vi "_MainOpenMV_New.vi"(11 "Port":string) -> (2 "Script Out":string)   [LabVIEW 2022 SP3]
uses:
  Processors.ctl
  _subs/CameraSetup.ctl
panel:
  in  "Make Main":bool
  out "ROI":T1={"left"=0, "top"=0, "right"=320, "bottom"=240}
  in  "Set ROI":bool
  out "roi":string
  in  "Set Threshold":bool
  in  "clear":bool
  out "Plots":T2
  out "Lab":string="[10,90,-40,40,-40,40]"
  out "Tx Buffer":string
  in  "Play":bool
  in  "Serial Port":string(combo)="ASRL30::INSTR"
  out "Version":string
  in  "Connect":bool
  out "FPS":dbl format="%#.2g"
  in  "Tabs":enum32{"Simple View", "REPL", "Python"}(tab)
  in  "Destination Info":enum32{"None", "UART", "SPI", "I2C", "WiFi"}(tab)
  in  "WiFi Info":T3={"WiFi"={"SSID"="", "Key"=""}, "SystemLink"={"APIKey"="", "Tag"="", "Type"="STRING"}}
  in  "Destination":enum16{"None", "UART", "SPI", "I2C", "WiFi"}(ring)
  out "Value":dbl(graph)
  in  "View":T4(ring)=enum."Nothing"
  in  "Params":T5(tab)
  in  "Color Statistic":u16(ring) items=["l_mean", "l_median", "l_mode", "l_sdev", "l_min", "l_max", "l_lower quartile", "l_upper quartile", "a_mean", "a_median", "a_mode", "a_sdev", "a_min", "a_max", "a_lq", "a_uq", "b_mean", "b_median", "b_mode", "b_sdev", "b_max", "b_min", "b_lq", "b_uq", "All statistics"]
  in  "Gray Statistic":u16(ring)=1 items=["mean", "median", "mode", "sdev", "min", "max", "lower quartile", "upper quartile", "All statistics"]
  in  "Blob Params":T6={"B[0]_Feature"=enum."# blobs", "Lab thresholds"="[10,90,-20,20,-20,20]", "Min Pixels"=100, "Min Area (box)"=100, "Merge"=TRUE, "Margin for merge"=10}
  in  "Face Parameter":u16(ring) items=["# faces", "All data"]
  in  "QR Return":u16(ring)=4 items=["x", "y", "w", "h", "payload", "version", "ecc_level", "mask", "data_type", "All data"]
  in  "Ctrl D":bool
  in  "Grab Script":bool
  in  "Line":u8(slide) scale=0.0..25.0
  in  "Send Line":bool
  out "Console":string
  in  "Notepad":string
  in  "Ctrl C":bool
  out "rows":string="  1\n  2\n  3\n  4\n  5\n  6\n  7\n  8\n  9\n 10\n 11\n 12\n 13\n 14\n 15\n 16\n 17\n 18\n 19\n 20\n 21\n"
  in  "Script":string="# Show Color - lmean\n\nimport sensor, image, time\n\nsensor.reset()\nsensor.set_pixformat(sensor.RGB565)\nsensor.set_framesize(sensor.QVGA)\nsensor.skip_frames(time = 2000)\n\nsensor.set_auto_gain(False)\nsensor.set_auto_whitebal(False) \n\nclock = time.clock()\n\n\n\nwhile(True):\n    clock.tick()\n    img = sensor.snapshot()\n    \n    print(img.statistics()[0])\n"
  in  "New":bool
  in  "Load":bool
  in  "Save":bool
  in  "File":path
  in  "startCode":string
  out "Size":string
  in  "stop":bool
  out "image":picture
  # "LabVIEW OpenMV"
  # "Note: i2c and SPI and WiFi are having issues"
  # "Use P4 for Tx and P5 for Rx and GND for ground\n\nDefault BAUD rate is 19200 - you can change this\nby editing the Python code (Python tab)"
  # "Use P0 for MOSI, P1 for MISO, P2 for SCLK, P3 for SS (active low)\n and GND for ground\n\nThe default is being an SPI slave - note that you can miss data\nin this mode"
  # "Use P4 for SCL and P5 for SDA and GND for ground\n\nThis runs as an i2c slave"
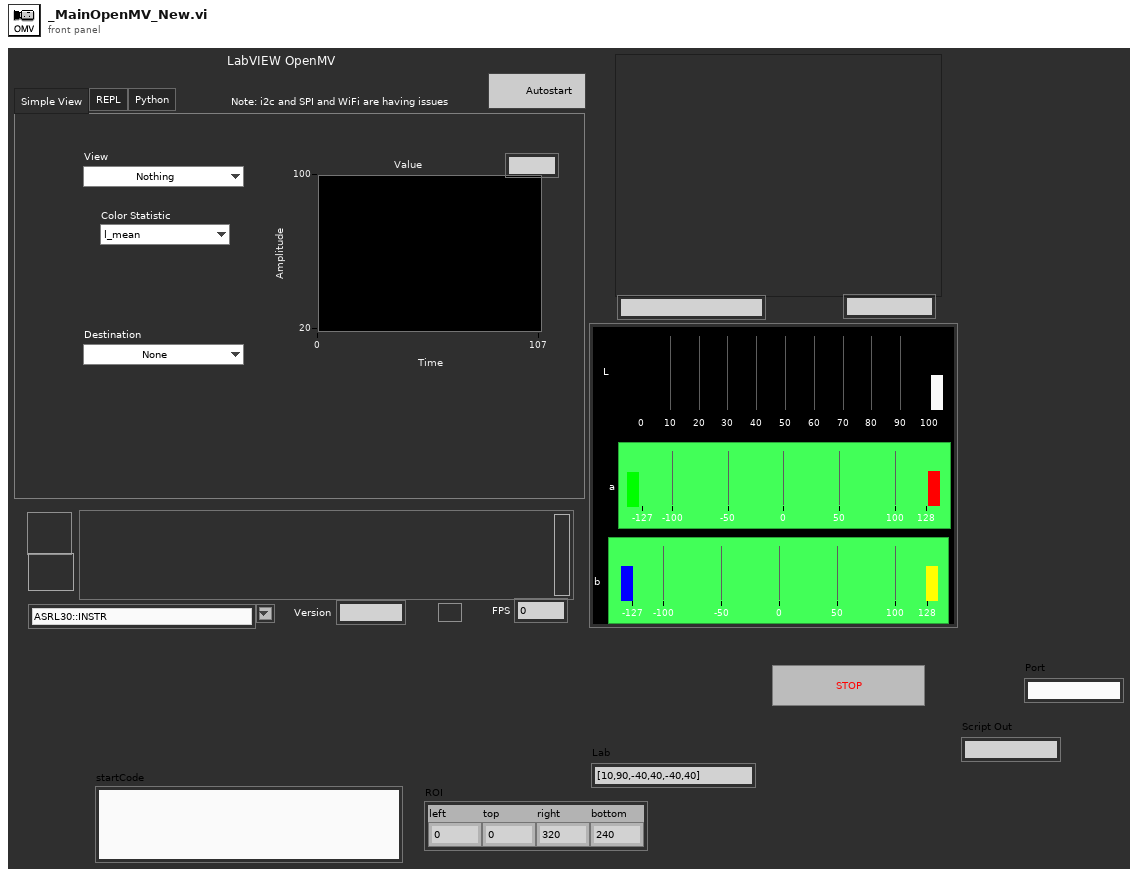
[diagram p1: front panel]
types:
  T1 = cluster{"left":i16, "top":i16, "right":i16, "bottom":i16}
  T2 = cluster{"L":dbl[], "a":cluster{i32, i32, dbl[]}, "b":cluster{i32, i32, dbl[]}}
  T3 = cluster{"WiFi":cluster{"SSID":string, "Key":string}, "SystemLink":cluster{"APIKey":string, "Tag":string, "Type":string}}
  T4 = enum16{"Color stats", "Nothing", "Greyscale stats", "Track Blobs", "Track Faces", "QRCode"}
  T5 = enum32{"C_ Stat", "G_Stats", "Blobs", "Face", "QR"}
  T6 = cluster{"B[0]_Feature":enum16{"x", "y", "width", "height", "pixels", "cx", "cy", "rotation", "code", "count", "# blobs", "All parameters"}, "Lab thresholds":string, "Min Pixels":i16, "Min Area (box)":i16, "Merge":bool, "Margin for merge":i16}
  T7 = typedef "Processors.ctl" = enum16{"SPIKE", "Pi", "Pi_ssh", "OpenMV", "Dunio"}
  T8 = enum8{"Enabled", "Disabled", "Disabled and Grayed Out"}
  T9 = enum16{"Color stats", "Greyscale stats", "Track Blobs", "Track Faces", "QRCode"}
  T10 = typedef "CameraSetup.ctl" = cluster{"Format":enum16{"GRAYSCALE", "RGB565", "BAYER"}, "size":enum16{"QQQQVGA (40x30)", "QQQVGA (80x60)", "QQVGA (160x120)", "QVGA (320x240)", "VGA (640x480)", "LCD (128x160)", "B64x32 (64x32)", "B64x64", "B128x64", "B128x128"}, "Skip frames (ms)":u16, "autoGain":bool, "autoWhitebal":bool}
  T11 = typedef "PythonCtrl.ctl" = cluster{"session":refnum<k35>, "PyPath":path, "Processor":T7, "Port":string, "version":string}
  T12 = typedef "imagedata.ctl" = cluster{"image type":i32, "image depth":i32, "image":u8[], "mask":u8[], "colors":u32[], "Rectangle":cluster{"left":i16, "top":i16, "right":i16, "bottom":i16}}
  T13 = typedef "Preferences.ctl" = cluster{"python":string, "arduino CLI":path, "pythonCodes":cluster{"pythonCode":path, "Color":u32}[], "FontSize":u8, "Text Colors":cluster{"Quote":u32, "function":u32, "Python":u32, "Comment":u32, "Triple Quote":u32, "Text":u32}, "SSH Logins":cluster{"IP Address":string, "Username":string, "password":string}[], "packet size":u8}
  T14 = cluster{"left":i32, "top":i32, "right":i32, "bottom":i32}
  T15 = typedef "eventvkey.ctl" = enum16{"ASCII", "Enter", "Return", "Shift", "Ctrl", "Alt", "Cmd", "Opt", "Caps", "NumLock", "Clear", "Break", "Up", "Down", "Left", "Right", "Insert", "Delete", "Home", "End", "PageUp", "PageDown", "Escape", "Help", "Pause", "ScrollLock", "F1", "F2", "F3", "F4", "F5", "F6", "F7", "F8", "F9", "F10", "F11", "F12", "F13", "F14", "F15", "F16", "F17", "F18", "F19", "F20", "F21", "F22", "F23", "F24", "Play", "VolumeUp", "VolumeDown", "Mute", "Two Byte Char"}
  T16 = cluster{"Shift":bool, "Ctrl":bool, "Alt":bool, "Cmd":bool, "Opt":bool}
  T17 = cluster{"Char":i16, "VKey":T15, "ScanCode":i16, "Mods":cluster{"Num Pad":bool, "Menu Key":bool}, "PlatMods":cluster{"Shift":bool, "Ctrl":bool, "Alt":bool, "Cmd":bool, "Opt":bool}, "FocusObj":refnum<vi>}
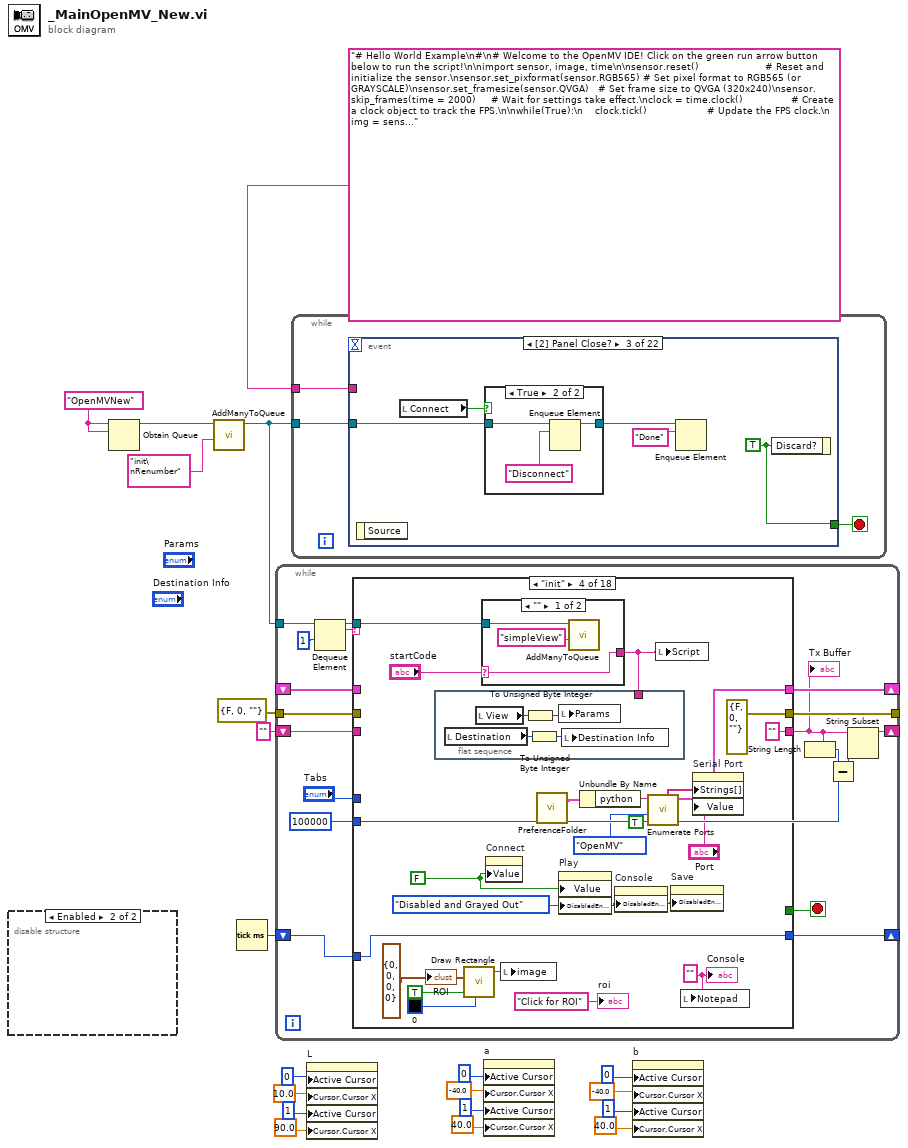
[diagram p0: block diagram]
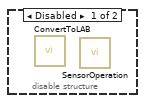
[diagram p2: hidden frame]
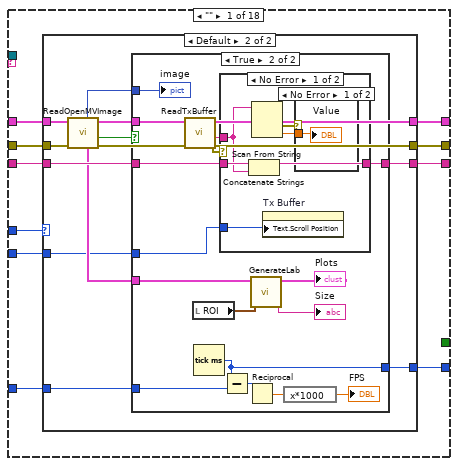
[diagram p3: hidden frame]
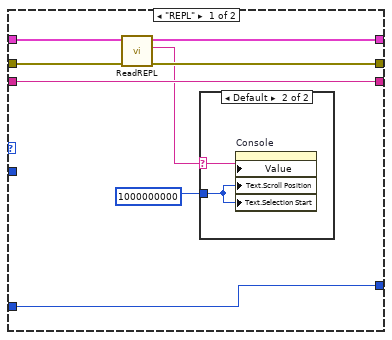
[diagram p4: hidden frame]
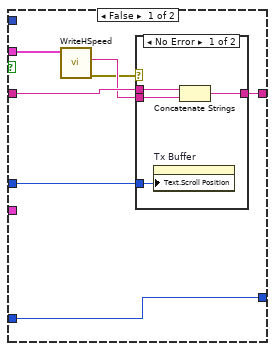
[diagram p6: hidden frame]
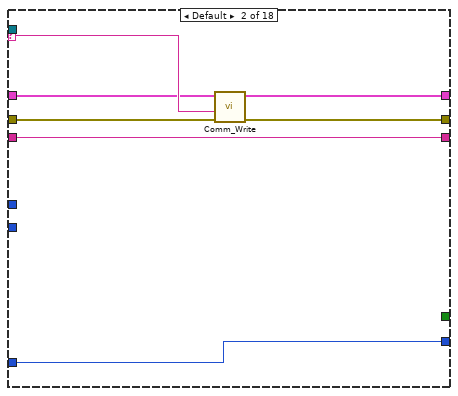
[diagram p10: hidden frame]
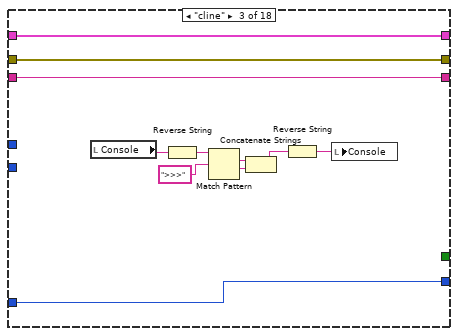
[diagram p11: hidden frame]
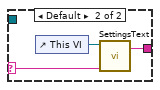
[diagram p12: hidden frame]
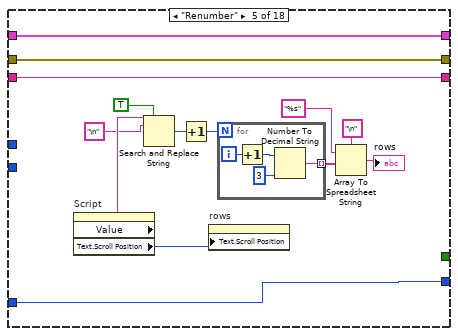
[diagram p13: hidden frame]
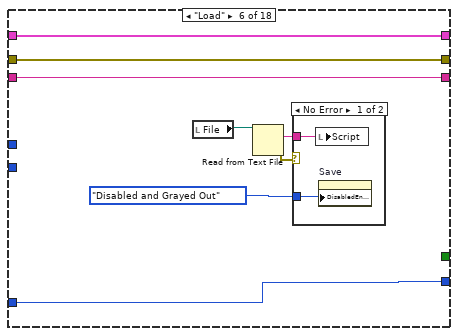
[diagram p14: hidden frame]
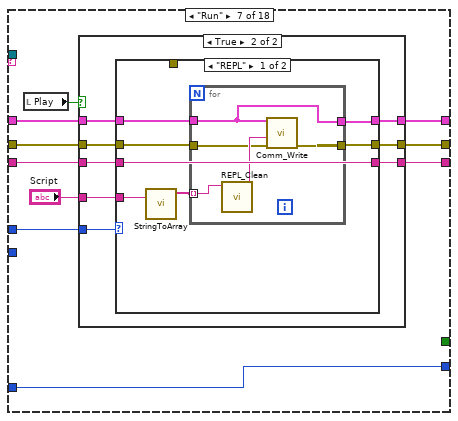
[diagram p16: hidden frame]
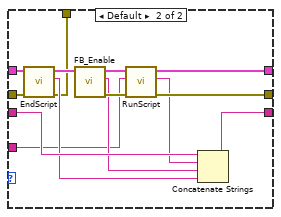
[diagram p18: hidden frame]
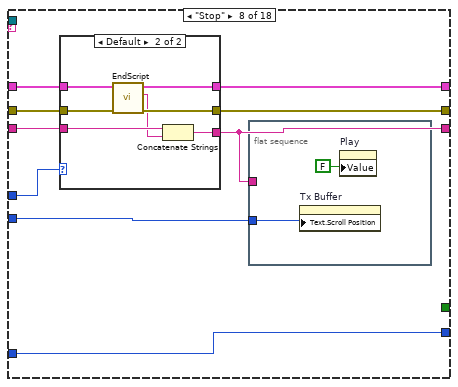
[diagram p19: hidden frame]
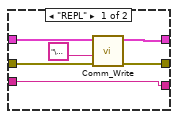
[diagram p20: hidden frame]
diagram:
  w20 = "OpenMVNew" ("name (unnamed)")
  n1 = disable-structure shown="Enabled" {
    frame Disabled {
      n2 = call "ConvertToLAB.vi"() -> ()  [unwired: 9 in, 3 out]
      n3 = call "SensorOperation.vi"() -> ()  [unwired: 11 in, 1 out]
    }
    frame Enabled {
    }
  }
  n4 = Obtain Queue(name (unnamed)=w20, element data type=w20) -> (queue out=w15:refnum<queue>)  [unwired: 3 in, 2 out]
  n5 = call "AddManyToQueue.vi"("Cmds"="init\nRenumber", "Queue in"=w15) -> ("Queue out"=w17:refnum<queue>)  [unwired: 9 in]
  n6 = Tick Count (ms)() -> (millisecond timer value=w18:u32)
  n7 = while {
    tunnel: w17 -> [w37]
    shift-right: [w34] -> _
    shift-left: _ -> [w35]
    shift-right: [w28] -> _
    shift-left: "" ("Tx Buffer") -> [w27]
    tunnel: errorcluster {"status"=FALSE, "code"=0, "source"=""} ("error out") -> [w32]
    tunnel: [w31] -> _
    shift-right: [w30] -> _
    shift-left: w18 -> [w29]
    stop <- w33 stop-if-true
    w25 = 100000 ("length (rest)")
    n8 = Dequeue Element(queue=w37, timeout in ms (-1)=1) -> (queue out=w21:refnum<queue>, element=w36:string)  [unwired: 1 in, 2 out]
    n9 = case shown="\"init\"" w36 {
      selector: w36 -> [_ w110 _ _ _ _ _ _ _ _ _ _ _ _ _ _ _ _]
      tunnel: w35 -> [w48 w107 w121 _ w168 w180 w192 w238 w261 w267 w307 w322 w346 w354 w366 w432 w437 w445]
      tunnel: [w45 w107 w121 w125 w168 w180 w190 w235 w258 w276 w298 w322 w346 w354 w366 w432 w437 w445] -> w34
      tunnel: [w46 w108 w120 errorcluster {"status"=FALSE, "code"=0, "source"=""} ("error out") w167 w179 w189 w236 w259 w275 w305 w321 w345 w353 w378 w431 w438 w444] -> w31
      tunnel: w32 -> [w47 w109 w120 _ w167 w179 w191 w237 w260 w274 w306 w321 w345 w353 w378 w431 w438 w444]
      tunnel: w27 -> [w44 w112 w123 _ w166 w178 w188 w233 w256 w273 w308 w320 w344 w352 w380 _ w435 w443]
      tunnel: [w43 w112 w123 "" ("Tx Buffer") w166 w178 w187 w231 w254 w273 w308 w320 w344 w352 w380 "" ("Tx Buffer") w434 w443] -> w24
      tunnel: [_ _ _ _ _ _ _ _ _ _ _ _ _ _ _ _ _ TRUE] -> w33
      tunnel: [w42 w111 w122 w142 w165 w177 w186 w234 w257 w272 w303 w318 w343 w351 w379 w433 w439 w441] -> w30
      tunnel: w29 -> [w41 w111 w122 w142 w165 w177 w186 w234 w257 w272 w303 w318 w343 w351 w379 w433 w439 w441]
      tunnel: w25 -> [w40 _ _ _ _ _ _ w232 w255 _ w299 _ _ _ _ _ _ _]
      tunnel: "Tabs" -> [w39 _ _ _ _ _ w184 w230 _ _ _ _ _ _ _ _ _ _]
      tunnel: w21 -> [_ _ _ w131 _ _ _ _ _ _ _ _ _ _ _ _ _ _]
      frame "" {
        n10 = case shown="Default" w39 {
          tunnel: w48 -> [w56 w68]
          tunnel: w47 -> [w55 w67]
          tunnel: [w53 w66] -> w46
          tunnel: [w54 w65] -> w45
          tunnel: w44 -> [w52 w64]
          tunnel: [w52 w63] -> w43
          tunnel: [w51 w62] -> w42
          tunnel: w41 -> [w51 w61]
          tunnel: w40 -> [_ w59]
          frame "REPL" {
            n11 = call "ReadREPL.vi"("error in (no error)"=w55, "Python"=w56) -> ("error out"=w53:errorcluster, "String"=w49:string, "Python"=w54:T11)  [unwired: 6 in, 1 out]
            n12 = case shown="Default" w49 {
              selector: w49 -> [_ w57]
              tunnel: u32 1000000000 ("Text.Selection:Start") -> [_ w58]
              frame "" {
              }
              frame Default {
                n13 = property on="Console" class="Str"("Value"=w57, "Text.Scroll Position"=w58, "Text.Selection Start"=w58) -> ()  [unwired: 2 in, 2 out]
              }
            }
          }
          frame Default {
            n14 = call "ReadOpenMVImage.vi"("error in"=w67, "Python"=w68) -> ("error out"=w66:errorcluster, "Good?"=w70:bool, "Python"=w65:T11, "image data"=w60:T12, "new picture"=w69:picture)  [unwired: 4 in, 1 out]
            n15 = case shown="True" w70 {
              tunnel: w69 -> [_ w92]
              tunnel: w65 -> [w73 w98]
              tunnel: [w75 w88] -> w63
              tunnel: w64 -> [w76 w86]
              tunnel: [w77 w97] -> w62
              tunnel: w61 -> [w77 w96]
              tunnel: w60 -> [_ w90]
              tunnel: w59 -> [w74 w83]
              frame False {
                n16 = call "WriteHSpeed.vi"("Python"=w73) -> ("error out"=w71:errorcluster, "read buffer"=w72:string)  [unwired: 8 in, 1 out]
                n17 = case shown="No Error" w71 {
                  tunnel: w72 -> [w81 _]
                  tunnel: w76 -> [w80 w82]
                  tunnel: [w79 w82] -> w75
                  tunnel: w74 -> [w78 _]
                  frame No Error {
                    n18 = property on="Tx Buffer" class="Str"("Text.Scroll Position"=w78) -> ()  [unwired: 2 in, 2 out]
                    n19 = Concatenate Strings(w80, w81) -> (w79:string)
                  }
                  frame Error {
                  }
                }
              }
              frame True {
                n20 = call "ReadTxBuffer.vi"("Python"=w98) -> ("error out"=w84:errorcluster, "Tx Buffer"=w85:string)  [unwired: 7 in, 2 out]
                n21 = local read "ROI"() -> (w89:T1)
                n22 = Tick Count (ms)() -> (millisecond timer value=w97:u32)
                n23 = case shown="No Error" w84 {
                  tunnel: [w104 w106] -> w88
                  tunnel: w86 -> [w101 w106]
                  tunnel: w85 -> [w100 _]
                  tunnel: w83 -> [w99 _]
                  frame No Error {
                    n24 = Concatenate Strings(w101, w100) -> (w104:string)
                    n25 = Scan From String(input string=w100) -> (error out=w103:errorcluster, output 1=w102:dbl)  [unwired: 4 in, 2 out]
                    n26 = property on="Tx Buffer" class="Str"("Text.Scroll Position"=w99) -> ()  [unwired: 2 in, 2 out]
                    n27 = case shown="No Error" w103 {
                      tunnel: w102 -> [w105 _]
                      frame No Error {
                        "Value" <- w105
                      }
                      frame Error {
                      }
                    }
                  }
                  frame Error {
                  }
                }
                n28 = Subtract(x=w97, y=w96) -> (x-y=w93:u32)
                n29 = Reciprocal(x=w93) -> (1/x=w95:dbl)
                n30 = call "GenerateLab.vi"("ROI"=w89, "image data"=w90) -> ("Dimensions"=→"Size":string, "Plots"=→"Plots":T2)  [unwired: 8 in]
                n31 = expression code="x*1000"(w95) -> (→"FPS":dbl)
                "image" <- w92
              }
            }
          }
        }
      }
      frame Default {
        n32 = call "Comm_Write.vi"("error in (no error)"=w109, "Text to write"=w110, "Python"=w107) -> ("error out"=w108:errorcluster)  [unwired: 7 in, 1 out]
      }
      frame "cline" {
        n33 = local read "Console"() -> (w113:string)
        n34 = Reverse String(1:w113) -> (0:w119:string)
        n35 = Match Pattern(string=w119, regular expression=">>>") -> (match substring=w116:string, after substring=w117:string)  [unwired: 1 in, 2 out]
        n36 = Concatenate Strings(w116, w117) -> (w115:string)
        n37 = Reverse String(1:w115) -> (0:w114:string)
        n38 = local write "Console"(w114) -> ()
      }
      frame "init" {
        w137 = "" ("Tx Buffer")
        w135 = T1 {"left"=0, "top"=0, "right"=0, "bottom"=0} ("rect")
        w136 = T8."Disabled and Grayed Out" ("Disabled")
        w138 = FALSE ("Connect")
        n39 = flat-sequence {
          tunnel: w132 -> [_]
          frame #0 {
            n40 = local read "Destination"() -> (w151:enum16{"None", "UART", "SPI", "I2C", "WiFi"})
            n41 = local read "View"() -> (w154:T4)
            n42 = To Unsigned Byte Integer(number=w154) -> (unsigned 8bit integer=w153:u8)
            n43 = To Unsigned Byte Integer(number=w151) -> (unsigned 8bit integer=w152:u8)
            n44 = local write "Params"(w153) -> ()
            n45 = local write "Destination Info"(w152) -> ()
          }
        }
        n46 = call <vilib>:"Draw Rectangle.vi"("rect"=w135, "fill?(F)"=TRUE, "color(black)"=u32 0) -> ("new picture"=w139:picture)  [unwired: 6 in]
        n47 = case shown="\"\"" "startCode" {
          selector: "startCode" -> [w147 w148]
          tunnel: [w147 w149] -> w132
          tunnel: w131 -> [w146 _]
          frame "" {
            n48 = call "AddManyToQueue.vi"("Cmds"="simpleView", "Queue in"=w146) -> ()  [unwired: 9 in, 1 out]
          }
          frame Default {
            n49 = control-ref of="This VI"() -> (w150:refnum<vi>)
            n50 = call "SettingsText.vi"("Saved code"=w148, "VI in"=w150) -> ("Python Code out"=w149:string)  [unwired: 8 in, 1 out]
          }
        }
        n51 = property on="Connect" class="Bool (strict)"("Value"=w138) -> ()  [unwired: 2 in, 2 out]
        n52 = local write "image"(w139) -> ()
        n53 = call "PreferenceFolder.vi"() -> ("Everything"=w126:T13)  [unwired: 4 in, 7 out]
        n54 = property on="Play" class="Bool (strict)"("Value"=w138, "DisabledEnum"=w136) -> ()  [unwired: 2 in, 2 out]
        n55 = Unbundle By Name(w126) -> ("python"=w129:string)
        n56 = property on="Console" class="Str"("DisabledEnum"=w136) -> ()  [unwired: 2 in, 2 out]
        n57 = call "Enumerate Ports.vi"("list?"=TRUE, "Processor"=Processors."OpenMV", "Python version"=w129) -> ("Python"=w125:T11, "possibilities"=w130:string[])  [unwired: 3 in, 4 out]
        n58 = local write "Script"(w132) -> ()
        n59 = property on="Save" class="Bool"("DisabledEnum"=w136) -> ()  [unwired: 2 in, 2 out]
        n60 = local write "Notepad"(w137) -> ()
        n61 = property on="Serial Port" class="CmbBox"("Strings[]"=w130, "Value"="Port") -> ()  [unwired: 2 in, 2 out]
        "Console" <- w137
        "roi" <- "Click for ROI" ("roi")
        "ROI" <- w135
      }
      frame "Renumber" {
        n62 = property on="Script" class="Str"() -> ("Value"=w164:string, "Text.Scroll Position"=w163:u32)  [unwired: 2 in, 2 out]
        n63 = Search and Replace String(replace all?=TRUE ("replace all? (F)"), input string=w164, search string="\n") -> (number of replacements=w162:i32)  [unwired: 5 in, 3 out]
        n64 = Increment(x=w162) -> (x+1=w155:i32)
        n65 = property on="rows" class="Str"("Text.Scroll Position"=w163) -> ()  [unwired: 2 in, 2 out]
        n66 = for {
          N: w155 -> [_]
          tunnel: [w172] -> w160 mode=indexing
          i -> [w169]
          n67 = Increment(x=w169) -> (x+1=w171:i32)
          n68 = Number To Decimal String(number=w171, width (-)=i16 3) -> (decimal integer string=w172:string)
        }
        n69 = Array To Spreadsheet String(delimiter (Tab)="\n", array=w160, 3:"%s" ("format string")) -> (spreadsheet string=→"rows":string)
      }
      frame "Load" {
        n70 = local read "File"() -> (w176:path)
        n71 = Read from Text File(file (use dialog)=w176) -> (text=w173:string, error out=w174:errorcluster)  [unwired: 3 in, 2 out]
        n72 = case shown="No Error" w174 {
          tunnel: T8."Disabled and Grayed Out" ("Disabled") -> [w182 _]
          tunnel: w173 -> [w181 _]
          frame No Error {
            n73 = local write "Script"(w181) -> ()
            n74 = property on="Save" class="Bool"("DisabledEnum"=w182) -> ()  [unwired: 2 in, 2 out]
          }
          frame Error {
          }
        }
      }
      frame "Run" {
        n75 = local read "Play"() -> (w185:bool)
        n76 = case shown="True" w185 {
          tunnel: w192 -> [w195 w203]
          tunnel: w191 -> [w194 w202]
          tunnel: [w195 w201] -> w190
          tunnel: [w194 w200] -> w189
          tunnel: w188 -> [w193 w198]
          tunnel: [w193 w199] -> w187
          tunnel: w184 -> [_ w197]
          tunnel: "Script" -> [_ w196]
          frame False {
          }
          frame True {
            n77 = case shown="\"REPL\"" w197 {
              tunnel: w203 -> [w209 w226]
              tunnel: w202 -> [w208 w225]
              tunnel: [w206 w224] -> w201
              tunnel: [w207 w223] -> w200
              tunnel: [w204 w222] -> w199
              tunnel: w198 -> [w204 w221]
              tunnel: w196 -> [w205 w217]
              tunnel: [_ w216] -> _
              frame "REPL" {
                n78 = call "StringToArray.vi"("write buffer"=w205) -> ("Array"=w210:string[])  [unwired: 10 in]
                n79 = for {
                  tunnel: w210 -> [w215] mode=indexing
                  tunnel: w209 -> [w211]
                  tunnel: w208 -> [w213]
                  tunnel: [w212] -> w207
                  tunnel: [w211] -> w206
                  n80 = call "REPL_Clean.vi"("Code in"=w215) -> ("Code cleaned"=w214:string)  [unwired: 10 in]
                  n81 = call "Comm_Write.vi"("error in (no error)"=w213, "Text to write"=w214, "Python"=w211) -> ("error out"=w212:errorcluster)  [unwired: 7 in, 1 out]
                }
              }
              frame Default {
                n82 = call "EndScript.vi"("error in (no error)"=w225, "Python"=w226) -> ("error out"=w216:errorcluster, "Tx for stopping code"=w218:string, "Python"=w229:T11)  [unwired: 7 in]
                n83 = call "FB_Enable.vi"("Python"=w229) -> ("error out"=w228:errorcluster, "Reply"=w219:string, "Python"=w227:T11)  [unwired: 8 in]
                n84 = call "RunScript.vi"("error in"=w228, "script"=w217, "Python"=w227) -> ("error out"=w223:errorcluster, "Tx"=w220:string, "Python"=w224:T11)  [unwired: 6 in]
                n85 = Concatenate Strings(w221, w220, w219, w218) -> (w222:string)
              }
            }
          }
        }
      }
      frame "Stop" {
        n86 = case shown="Default" w230 {
          tunnel: w238 -> [w239 w250]
          tunnel: w237 -> [w242 w249]
          tunnel: [w240 w248] -> w236
          tunnel: [w239 w247] -> w235
          tunnel: w233 -> [w243 w246]
          tunnel: [w243 w244] -> w231
          frame "REPL" {
            n87 = call "Comm_Write.vi"("error in (no error)"=w242, "Text to write"="\u0003" ("write buffer"), "Python"=w239) -> ("error out"=w240:errorcluster)  [unwired: 7 in, 1 out]
          }
          frame Default {
            n88 = call "EndScript.vi"("error in (no error)"=w249, "Python"=w250) -> ("error out"=w248:errorcluster, "Tx for stopping code"=w245:string, "Python"=w247:T11)  [unwired: 7 in]
            n89 = Concatenate Strings(w246, w245) -> (w244:string)
          }
        }
        n90 = flat-sequence {
          tunnel: w232 -> [w252]
          tunnel: w231 -> [_]
          frame #0 {
            n91 = property on="Tx Buffer" class="Str"("Text.Scroll Position"=w252) -> ()  [unwired: 2 in, 2 out]
            n92 = property on="Play" class="Bool (strict)"("Value"=FALSE ("Play")) -> ()  [unwired: 2 in, 2 out]
          }
        }
      }
      frame "stopForREPL" {
        n93 = call "EndScript.vi"("error in (no error)"=w260, "Python"=w261) -> ("error out"=w259:errorcluster, "Tx for stopping code"=w253:string, "Python"=w258:T11)  [unwired: 7 in]
        n94 = Concatenate Strings(w256, w253) -> (w254:string)
        n95 = flat-sequence {
          tunnel: w255 -> [w263]
          tunnel: w254 -> [_]
          frame #0 {
            n96 = property on="Tx Buffer" class="Str"("Text.Scroll Position"=w263) -> ()  [unwired: 2 in, 2 out]
            n97 = property on="Play" class="Bool (strict)"("Value"=FALSE ("Play")) -> ()  [unwired: 2 in, 2 out]
          }
        }
      }
      frame "Connect" {
        n98 = local read "Tabs"() -> (w269:enum32{"Simple View", "REPL", "Python"})
        n99 = Match Pattern(string="Serial Port", regular expression=":") -> (before substring=w265:string)  [unwired: 1 in, 3 out]
        n100 = Not Equal?(x=w269, y=enum32{"Simple View", "REPL", "Python"}."REPL") -> (x != y?=w271:bool)
        n101 = call "HighSpeedInit.vi"("error in"=w274, "Port"=w265, "Fast"=w271, "Python"=w267) -> ("error out"=w268:errorcluster, "Python"=w277:T11)  [unwired: 6 in]
        n102 = case shown="Error" w268 {
          selector: w268 -> [w278 w297]
          tunnel: w277 -> [w283 w294]
          tunnel: [w282 w294] -> w276
          tunnel: [w281 w297] -> w275
          tunnel: w269 -> [w280 _]
          frame No Error {
            w279 = T8."Enabled" ("Disabled")
            n103 = property on="Play" class="Bool (strict)"("DisabledEnum"=w279) -> ()  [unwired: 2 in, 2 out]
            n104 = case shown="\"REPL\"" w280 {
              tunnel: w278 -> [w287 w293]
              tunnel: w283 -> [w285 w292]
              tunnel: [w285 w290] -> w282
              tunnel: [w286 w289] -> w281
              tunnel: w279 -> [w288 _]
              frame "REPL" {
                n105 = property on="Console" class="Str"("DisabledEnum"=w288) -> ()  [unwired: 2 in, 2 out]
                n106 = call "Comm_Write.vi"("error in (no error)"=w287, "Text to write"="\n\n" ("write buffer"), "Python"=w285) -> ("error out"=w286:errorcluster)  [unwired: 7 in, 1 out]
              }
              frame Default {
                n107 = call "AskVersion.vi"("error in"=w293, "Python"=w292) -> ("error out"=w289:errorcluster, "Version"=→"Version":string, "Python"=w290:T11)  [unwired: 7 in]
              }
            }
          }
          frame Error {
            n108 = local write "Connect"(FALSE ("Connect")) -> ()
            n109 = One Button Dialog(message="Cannot initialize port. Try another") -> ()  [unwired: 1 in, 1 out]
          }
        }
      }
      frame "Disconnect" {
        w300 = T8."Disabled and Grayed Out" ("Disabled")
        n110 = local read "Tabs"() -> (w301:enum32{"Simple View", "REPL", "Python"})
        n111 = property on="Tx Buffer" class="Str"("Text.Scroll Position"=w299) -> ()  [unwired: 2 in, 2 out]
        n112 = case shown="Default" w301 {
          tunnel: [w310 w314] -> w298
          tunnel: w307 -> [w310 w313]
          tunnel: w306 -> [w309 w312]
          tunnel: [w309 w311] -> w305
          frame "REPL" {
          }
          frame Default {
            n113 = call "EndScript.vi"("error in (no error)"=w312, "Python"=w313) -> ("error out"=w311:errorcluster, "Python"=w314:T11)  [unwired: 7 in, 1 out]
          }
        }
        n114 = call "CloseHS.vi"("error in (no error)"=w305, "Python"=w298) -> ()  [unwired: 10 in]
        n115 = local write "Connect"(FALSE ("Connect")) -> ()
        n116 = property on="Play" class="Bool (strict)"("Value"=FALSE ("Play"), "DisabledEnum"=w300) -> ()  [unwired: 2 in, 2 out]
        n117 = property on="Console" class="Str"("DisabledEnum"=w300) -> ()  [unwired: 2 in, 2 out]
      }
      frame "ROI" {
        n118 = local read "image"() -> (w319:picture)
        n119 = local read "ROI"() -> (w315:T1)
        n120 = call "OpenMV_SelectROI.vi"("ROI"=w315, "image"=w319) -> ("Rect"=w317:T14)  [unwired: 1 in]
        n121 = local write "ROI"(w317) -> ()
        n122 = call "ROIText.vi"("ROI"=w317) -> ("r"=w316:string)  [unwired: 7 in, 3 out]
        n123 = local write "roi"(w316) -> ()
      }
      frame "Lab" {
        n124 = property on="L" class="WFGraph (strict)"("Active Cursor"=u32 0, "Active Cursor"=u32 1) -> ("Cursor.Cursor X"=w336:dbl, "Cursor.Cursor X"=w335:dbl)  [unwired: 2 in, 2 out]
        n125 = property on="a" class="WFGraph (strict)"("Active Cursor"=u32 0, "Active Cursor"=u32 1) -> ("Cursor.Cursor X"=w337:dbl, "Cursor.Cursor X"=w338:dbl)  [unwired: 2 in, 2 out]
        n126 = property on="b" class="WFGraph (strict)"("Active Cursor"=u32 0, "Active Cursor"=u32 1) -> ("Cursor.Cursor X"=w339:dbl, "Cursor.Cursor X"=w340:dbl)  [unwired: 2 in, 2 out]
        n127 = Max & Min(x=w336, y=w335) -> (max(x,y)=w328:dbl, min(x,y)=w327:dbl)
        n128 = Max & Min(x=w337, y=w338) -> (max(x,y)=w326:dbl, min(x,y)=w325:dbl)
        n129 = Max & Min(x=w339, y=w340) -> (max(x,y)=w323:dbl, min(x,y)=w324:dbl)
        n130 = Format Into String(format string="[%d,%d,%d,%d,%d,%d]", w327, w328, w325, w326, w324, w323) -> (resulting string=→"Lab":string)  [unwired: 2 in, 1 out]
      }
      frame "LabPopup" {
        n131 = local read "image"() -> (w349:picture)
        n132 = local read "ROI"() -> (w347:T1)
        n133 = call "OpenMV_SelectLab.vi"("ROI"=w347, "image"=w349) -> ("ROI out"=w348:T14, "thresholds"=w350:dbl[])
        n134 = for {
          tunnel: w350 -> [w355] mode=indexing
          i -> [w359]
          n135 = Quotient & Remainder(x=w359, y=2) -> (x-y*floor(x/y)=w356:i32, floor(x/y)=w357:i32)
          n136 = case shown="0" w357 {
            tunnel: w356 -> [_ w361 w363 w365]
            tunnel: w355 -> [_ w360 w362 w364]
            frame Default {
            }
            frame 0 {
              n137 = property on="L" class="WFGraph (strict)"("Active Cursor"=w361, "Cursor.Cursor X"=w360) -> ()  [unwired: 2 in, 2 out]
            }
            frame 1 {
              n138 = property on="a" class="WFGraph (strict)"("Active Cursor"=w363, "Cursor.Cursor X"=w362) -> ()  [unwired: 2 in, 2 out]
            }
            frame 2 {
              n139 = property on="b" class="WFGraph (strict)"("Active Cursor"=w365, "Cursor.Cursor X"=w364) -> ()  [unwired: 2 in, 2 out]
            }
          }
        }
        n140 = local write "ROI"(w348) -> ()
      }
      frame "simpleView" {
        n141 = local read "ROI"() -> (w373:T1)
        n142 = local read "Lab"() -> (w372:string)
        n143 = case shown="\"Nothing\"" "View" {
          tunnel: "Destination" -> [w388 _ w401 w411 w419 w427]
          tunnel: [w387 "import sensor, image, time\n\nsensor.reset()               \nsensor.set_pixformat(sensor.RGB565) \nsensor.set_framesize(sensor.QVGA)  \nsensor.skip_frames(time = 2000)     # Wait for settings take effect.\nclock = time.clock()                # Create a clock object to track the FPS.\n\nwhile(True):\n    clock.tick()                               # Update the FPS clock.\n    img = sensor.snapshot()         # Take a picture and return the image.\n    print(clock.fps())              \n" ("Python Code") w400 w410 w417 w425] -> w370
          tunnel: "WiFi Info" -> [w386 _ w399 w409 w418 w426]
          tunnel: w373 -> [w385 _ w398 w404 w415 w423]
          tunnel: w372 -> [_ _ _ w406 _ _]
          tunnel: [w384 _ w397 w405 w416 w424] -> _
          tunnel: w366 -> [w381 _ w390 w402 w412 w420]
          frame "Color stats", Default {
            n144 = call "simpleStatistics.vi"("WiFi Info"=w386, "ROI"=w385, "Output"=w388, "Camera Setup"=T10 {"Format"=enum."RGB565", "size"=enum."QVGA (320x240)", "Skip frames (ms)"=2000, "autoGain"=TRUE, "autoWhitebal"=TRUE}, "Statistic"="Color Statistic", "Python"=w381) -> ("error out"=w384:errorcluster, "Python Code"=w387:string)  [unwired: 3 in, 1 out]
          }
          frame "Nothing" {
          }
          frame "Greyscale stats" {
            n145 = Not Equal?(x="Gray Statistic", y=u8 8) -> (x != y?=w395:bool)
            n146 = Select(t="Gray Statistic", s=w395, f=u8 24 ("y")) -> (s? t:f=w394:u16)
            n147 = call "simpleStatistics.vi"("WiFi Info"=w399, "ROI"=w398, "Output"=w401, "Camera Setup"=T10 {"Format"=enum."GRAYSCALE", "size"=enum."QVGA (320x240)", "Skip frames (ms)"=2000, "autoGain"=TRUE, "autoWhitebal"=TRUE}, "Statistic"=w394, "Python"=w390) -> ("error out"=w397:errorcluster, "Python Code"=w400:string)  [unwired: 3 in, 1 out]
          }
          frame "Track Blobs" {
            n148 = Bundle By Name(cluster="Blob Params", "Lab thresholds"=w406) -> (w407:T6)
            n149 = call "trackBlobs.vi"("WiFi Info"=w409, "ROI"=w404, "Output"=w411, "Camera Setup"=T10 {"Format"=enum."RGB565", "size"=enum."QVGA (320x240)", "Skip frames (ms)"=2000, "autoGain"=TRUE, "autoWhitebal"=TRUE}, "Blob Params"=w407, "Python"=w402) -> ("error out"=w405:errorcluster, "Python Code"=w410:string)  [unwired: 3 in, 1 out]
          }
          frame "QRCode" {
            n150 = call "QRCodes.vi"("WiFi Info"=w418, "ROI"=w415, "Output"=w419, "Camera Setup"=T10 {"Format"=enum."RGB565", "size"=enum."QVGA (320x240)", "Skip frames (ms)"=2000, "autoGain"=FALSE, "autoWhitebal"=FALSE}, "Value"="QR Return", "Python"=w412) -> ("error out"=w416:errorcluster, "Python Code"=w417:string)  [unwired: 3 in, 1 out]
          }
          frame "Track Faces" {
            n151 = call "trackFaces.vi"("WiFi Info"=w426, "ROI"=w423, "Output"=w427, "Camera Setup"=T10 {"Format"=enum."GRAYSCALE", "size"=enum."QVGA (320x240)", "Skip frames (ms)"=2000, "autoGain"=FALSE, "autoWhitebal"=FALSE}, "Value"="Face Parameter", "Python"=w420) -> ("error out"=w424:errorcluster, "Python Code"=w425:string)  [unwired: 3 in, 1 out]
          }
        }
        n152 = Equal?(x=T9."Track Blobs" ("View"), y="View") -> (x = y?=w377:bool)
        n153 = for {
          N: 2 -> [_]
          tunnel: w377 -> [w429]
          i -> [w428]
          n154 = property on="L" class="WFGraph (strict)"("Active Cursor"=w428, "Cursor.Visible"=w429) -> ()  [unwired: 2 in, 2 out]
          n155 = property on="a" class="WFGraph (strict)"("Active Cursor"=w428, "Cursor.Visible"=w429) -> ()  [unwired: 2 in, 2 out]
          n156 = property on="b" class="WFGraph (strict)"("Active Cursor"=w428, "Cursor.Visible"=w429) -> ()  [unwired: 2 in, 2 out]
        }
        n157 = control-ref of="This VI"() -> (w369:refnum<vi>)
        n158 = call "SettingsText.vi"("Python Code in"=w370, "VI in"=w369) -> ("Python Code out"=w367:string)  [unwired: 8 in, 1 out]
        n159 = local write "Script"(w367) -> ()
      }
      frame "Clear" {
      }
      frame "Main.py" {
        n160 = local read "Script"() -> (w436:string)
        n161 = call "OMV_UploadMainPY.vi"("Script"=w436, "Tx Buffer"=w435, "Python"=w437) -> ("Tx Buffer Out"=w434:string)  [unwired: 8 in]
      }
      frame "Done" {
        n162 = local read "Script"() -> (→"Script Out":string)
      }
    }
    "Tx Buffer" <- w24
    n163 = String Length(string=w24) -> (length=w26:i32)
    n164 = Subtract(x=w26, y=w25) -> (x-y=w23:i32)
    n165 = String Subset(string=w24, offset (0)=w23) -> (substring=w28:string)  [unwired: 1 in]
  }
  n166 = while {
    tunnel: w17 -> [w447]
    tunnel: "# Hello World Example\n#\n# Welcome to the OpenMV IDE! Click on the green run arrow button below to run the script!\n\nimport sensor, image, time\n\nsensor.reset()                      # Reset and initialize the sensor.\nsensor.set_pixformat(sensor.RGB565) # Set pixel format to RGB565 (or GRAYSCALE)\nsensor.set_framesize(sensor.QVGA)   # Set frame size to QVGA (320x240)\nsensor.skip_frames(time = 2000)     # Wait for settings take effect.\nclock = time.clock()                # Create a clock object to track the FPS.\n\nwhile(True):\n    clock.tick()                    # Update the FPS clock.\n    img = sensor.snapshot()         # Take a picture and return the image.\n    print(clock.fps())              # Note: OpenMV Cam runs about half as fast when connected\n                                    # to the IDE. The FPS should increase once disconnected.\n" ("startCode") -> [w446]
    stop <- w448 stop-if-true
    n167 = event shown="[2] Panel Close?" {
      selector: _ -> [_ _ _ _ _ _ _ _ _ _ _ _ _ _ _ _ _ _ _ _ _ _]
      dyn-events: _ -> [_ _ _ _ _ _ _ _ _ _ _ _ _ _ _ _ _ _ _ _ _ _]
      timeout: _ -> [_ _ _ _ _ _ _ _ _ _ _ _ _ _ _ _ _ _ _ _ _ _]
      tunnel: [_ "stop" w458 _ _ _ _ _ _ _ _ _ _ _ _ _ _ _ _ _ _ _] -> w448
      tunnel: w447 -> [_ w451 w461 w470 w479 w484 w486 _ w494 _ w518 w525 w529 w532 w535 w538 w540 _ w551 _ w556 w562]
      tunnel: w446 -> [_ _ _ _ _ _ _ w490 _ _ _ _ _ _ _ _ _ _ _ _ _ _]
      event Timeout {
        n168 = event-data() -> ()  [unwired: 1 in, 1 out]
      }
      event "stop": Value Change {
        n169 = event-data() -> ()  [unwired: 1 in, 1 out]
        n170 = local read "Connect"() -> (w449:bool)
        n171 = case shown="True" w449 {
          tunnel: w451 -> [w454 w457]
          tunnel: [w454 w456] -> w450
          frame False {
          }
          frame True {
            n172 = Enqueue Element(queue=w457, element="Disconnect") -> (queue out=w456:refnum<queue>)  [unwired: 2 in, 2 out]
          }
        }
        n173 = Enqueue Element(queue=w450, element="Done") -> ()  [unwired: 2 in, 3 out]
      }
      event Panel Close? {
        w458 = TRUE ("Discard?")
        n174 = event-data() -> ()  [unwired: 1 in, 1 out]
        n175 = local read "Connect"() -> (w459:bool)
        n176 = case shown="True" w459 {
          tunnel: w461 -> [w463 w466]
          tunnel: [w463 w465] -> w460
          frame False {
          }
          frame True {
            n177 = Enqueue Element(queue=w466, element="Disconnect") -> (queue out=w465:refnum<queue>)  [unwired: 2 in, 2 out]
          }
        }
        n178 = Enqueue Element(queue=w460, element="Done") -> ()  [unwired: 2 in, 3 out]
        n179 = event-data("Discard?"=w458) -> ()  [unwired: 1 in, 1 out]
      }
      event "Tabs": Value Change {
        n180 = event-data() -> ("NewVal"=w467:enum32{"Simple View", "REPL", "Python"})  [unwired: 1 in]
        n181 = case shown="\"REPL\"" w467 {
          tunnel: w470 -> [w471 w473]
          tunnel: [w471 w472] -> w469
          frame Default {
          }
          frame "REPL" {
            n182 = call "AddManyToQueue.vi"("Cmds"="stopForREPL\nDisconnect", "Queue in"=w473) -> ("Queue out"=w472:refnum<queue>)  [unwired: 9 in]
          }
        }
        n183 = Enqueue Element(queue=w469, element="Renumber") -> ()  [unwired: 2 in, 3 out]
      }
      event "Play": Value Change {
        n184 = event-data() -> ()  [unwired: 1 in, 1 out]
        n185 = Select(t="Run" ("element"), s="Play", f="Stop" ("element")) -> (s? t:f=w475:string)
        n186 = Enqueue Element(queue=w479, element=w475) -> ()  [unwired: 2 in, 3 out]
      }
      event "Connect": Value Change {
        n187 = event-data() -> ()  [unwired: 1 in, 1 out]
        n188 = Select(t="Connect" ("element"), s="Connect", f="Disconnect" ("element")) -> (s? t:f=w482:string)
        n189 = Enqueue Element(queue=w484, element=w482) -> ()  [unwired: 2 in, 3 out]
      }
      event "Script": Value Change {
        n190 = event-data() -> ()  [unwired: 1 in, 1 out]
        n191 = Enqueue Element(queue=w486, element="Renumber") -> ()  [unwired: 2 in, 3 out]
        n192 = property on="Save" class="Bool"("DisabledEnum"=T8."Enabled" ("Disabled")) -> ()  [unwired: 2 in, 2 out]
      }
      event "New": Value Change {
        n193 = event-data() -> ()  [unwired: 1 in, 1 out]
        n194 = property on="Save" class="Bool"() -> ("DisabledEnum"=w489:T8)  [unwired: 2 in, 2 out]
        n195 = call "CheckReplace.vi"("DisabledEnum"=w489) -> ("Replace?"=w488:bool)  [unwired: 10 in]
        n196 = case shown="True" w488 {
          tunnel: w490 -> [_ w492]
          frame False {
          }
          frame True {
            n197 = property on="Save" class="Bool"("DisabledEnum"=T8."Enabled" ("Disabled")) -> ()  [unwired: 2 in, 2 out]
            n198 = local write "Script"(w492) -> ()
            n199 = local write "File"(path "" ("File")) -> ()
          }
        }
      }
      event "Load", "File": Value Change {
        n200 = event-data() -> ()  [unwired: 1 in, 1 out]
        n201 = property on="Save" class="Bool"() -> ("DisabledEnum"=w496:T8)  [unwired: 2 in, 2 out]
        n202 = call "CheckReplace.vi"("DisabledEnum"=w496) -> ("Replace?"=w495:bool)  [unwired: 10 in]
        n203 = case shown="True" w495 {
          tunnel: w494 -> [_ w499]
          frame False {
          }
          frame True {
            n204 = call "File Dialog2"() -> ("selected path"=w498:path, "cancelled"=w497:bool)  [unwired: 12 in, 2 out]
            n205 = case shown="False" w497 {
              tunnel: w499 -> [w501 _]
              tunnel: w498 -> [w500 _]
              frame False {
                n206 = local write "File"(w500) -> ()
                n207 = Enqueue Element(queue=w501, element="Load") -> (queue out=w502:refnum<queue>)  [unwired: 2 in, 2 out]
                n208 = Enqueue Element(queue=w502, element="Renumber") -> ()  [unwired: 2 in, 3 out]
              }
              frame True {
              }
            }
          }
        }
      }
      event "Save": Value Change {
        n209 = event-data() -> ()  [unwired: 1 in, 1 out]
        n210 = Empty String/Path?(string/path="File") -> (empty?=w507:bool)
        n211 = case shown="True" w507 {
          tunnel: [w511 w513] -> w510
          tunnel: "File" -> [w511 _]
          tunnel: [_ w512] -> w505
          frame False {
          }
          frame True {
            n212 = call "File Dialog2"() -> ("selected path"=w513:path, "cancelled"=w512:bool)  [unwired: 12 in, 2 out]
          }
        }
        n213 = local read "Script"() -> (w509:string)
        n214 = case shown="False" w505 {
          tunnel: w510 -> [w516 _]
          tunnel: w509 -> [w515 _]
          tunnel: T8."Disabled and Grayed Out" ("Disabled") -> [w514 _]
          frame False {
            n215 = Write to Text File(file (use dialog)=w516, text=w515) -> ()  [unwired: 2 in, 3 out]
            n216 = property on="Save" class="Bool"("DisabledEnum"=w514) -> ()  [unwired: 2 in, 2 out]
          }
          frame True {
          }
        }
      }
      event "View", "Destination", "Color Statistic", "Gray Statistic", "Blob Params", "QR Return", "Params", "Face Parameter": Value Change {
        n217 = event-data() -> ()  [unwired: 1 in, 1 out]
        n218 = call "AddManyToQueue.vi"("Cmds"="Stop\nsimpleView\nRun", "Queue in"=w518) -> ()  [unwired: 9 in, 1 out]
        n219 = local read "Destination"() -> (w519:enum16{"None", "UART", "SPI", "I2C", "WiFi"})
        n220 = local read "View"() -> (w522:T4)
        n221 = To Unsigned Byte Integer(number=w522) -> (unsigned 8bit integer=w521:u8)
        n222 = To Unsigned Byte Integer(number=w519) -> (unsigned 8bit integer=w520:u8)
        n223 = local write "Params"(w521) -> ()
        n224 = local write "Destination Info"(w520) -> ()
      }
      event "Set ROI": Value Change {
        n225 = event-data() -> ()  [unwired: 1 in, 1 out]
        n226 = local read "Tabs"() -> (w523:enum32{"Simple View", "REPL", "Python"})
        n227 = case shown="Default" w523 {
          tunnel: ["Stop\nROI\nsimpleView\nRenumber\nRun" "Stop\nROI\nRun"] -> w524
          frame "Simple View" {
          }
          frame Default {
          }
        }
        n228 = call "AddManyToQueue.vi"("Cmds"=w524, "Queue in"=w525) -> ()  [unwired: 9 in, 1 out]
      }
      event "Plots.L", "Plots.a", "Plots.b": Cursor Move {
        n229 = event-data() -> ()  [unwired: 1 in, 1 out]
        n230 = call "AddManyToQueue.vi"("Cmds"="Stop\nLab\nsimpleView\nRenumber\nRun", "Queue in"=w529) -> ()  [unwired: 9 in, 1 out]
      }
      event "Set Threshold": Value Change {
        n231 = event-data() -> ()  [unwired: 1 in, 1 out]
        n232 = local read "Tabs"() -> (w530:enum32{"Simple View", "REPL", "Python"})
        n233 = case shown="Default" w530 {
          tunnel: ["Stop\nLabPopup\nLab\nsimpleView\nRenumber\nRun" "Stop\nLabPopup\nLab\nRun"] -> w531
          frame "Simple View" {
          }
          frame Default {
          }
        }
        n234 = call "AddManyToQueue.vi"("Cmds"=w531, "Queue in"=w532) -> ()  [unwired: 9 in, 1 out]
      }
      event "clear": Value Change {
        n235 = event-data() -> ()  [unwired: 1 in, 1 out]
        n236 = Enqueue Element(queue=w535, element="Clear") -> ()  [unwired: 2 in, 3 out]
      }
      event "Ctrl C": Value Change {
        n237 = event-data() -> ()  [unwired: 1 in, 1 out]
        n238 = call "AddManyToQueue.vi"("Cmds"="\u0003" ("write buffer"), "Queue in"=w538) -> ()  [unwired: 9 in, 1 out]
      }
      event "Ctrl D": Value Change {
        n239 = event-data() -> ()  [unwired: 1 in, 1 out]
        n240 = call "AddManyToQueue.vi"("Cmds"="\u0004" ("write buffer"), "Queue in"=w540) -> ()  [unwired: 9 in, 1 out]
      }
      event "Line": Value Change {
        n241 = event-data() -> ()  [unwired: 1 in, 1 out]
        n242 = property on="Notepad" class="Str"() -> ("Text.Text"=w546:string)  [unwired: 2 in, 2 out]
        n243 = call "Select.vi"("Line"="Line", "Text.Text"=w546) -> ("scale"=w543:i32, "Text min"=w541:i32, "Text max"=w542:i32)  [unwired: 7 in]
        n244 = property on="Line" class="Slide (strict)"("Scale.Maximum"=w543) -> ()  [unwired: 2 in, 2 out]
        n245 = property on="Notepad" class="Str"("Key Focus"=TRUE, "Text.Selection End"=w542, "Text.Selection Start"=w541) -> ()  [unwired: 2 in, 2 out]
      }
      event "Send Line": Value Change {
        n246 = event-data() -> ()  [unwired: 1 in, 1 out]
        n247 = local read "Line"() -> (w549:u8)
        n248 = call "StringToArray.vi"("write buffer"="Notepad") -> ("Array"=w552:string[])  [unwired: 10 in]
        n249 = Index Array(array=w552, index=w549) -> (element=w547:string)
        n250 = call "REPL_Clean.vi"("Code in"=w547) -> ("Code cleaned"=w550:string)  [unwired: 10 in]
        n251 = Enqueue Element(queue=w551, element=w550) -> ()  [unwired: 2 in, 3 out]
        n252 = Increment(x=w549) -> (x+1=w548:u8)
        n253 = property on="Line" class="Slide (strict)"("Val(Sgnl)"=w548) -> ()  [unwired: 2 in, 2 out]
      }
      event "Grab Script": Value Change {
        w554 = u8 0 ("Line")
        n254 = event-data() -> ()  [unwired: 1 in, 1 out]
        n255 = property on="Line" class="Slide (strict)"("Val(Sgnl)"=w554) -> ()  [unwired: 2 in, 2 out]
        n256 = local read "Script"() -> (w555:string)
        n257 = property on="Notepad" class="Str"("Value"=w555, "Text.Scroll Position"=w554) -> ()  [unwired: 2 in, 2 out]
      }
      event "Make Main": Value Change {
        n258 = event-data() -> ()  [unwired: 1 in, 1 out]
        n259 = call "AddManyToQueue.vi"("Cmds"="Stop\nMain.py", "Queue in"=w556) -> ()  [unwired: 9 in, 1 out]
      }
      event Key Down? {
        n260 = event-data() -> ("Char"=w568:i16, "VKey"=w567:T15, "ScanCode"=w566:i16, "Mods"=w565:cluster{"Num Pad":bool, "Menu Key":bool}, "PlatMods"=w564:T16, "FocusObj"=w561:refnum<vi>)  [unwired: 1 in]
        n261 = control-ref of="Console"() -> (w559:refnum<vi>)
        n262 = Bundle("Char"=w568, "VKey"=w567, "ScanCode"=w566, "Mods"=w565, "PlatMods"=w564, "FocusObj"=w561) -> (w560:T17)  [unwired: 1 in]
        n263 = Equal?(x=w561, y=w559) -> (x = y?=w563:bool)
        n264 = case shown="True" w563 {
          tunnel: w560 -> [_ w574]
          tunnel: w562 -> [_ w572]
          tunnel: [_ TRUE] -> w558
          frame False {
          }
          frame True {
            n265 = call "KeyboardCalls.vi"("Cluster"=w574) -> ("Extras"=w570:enum16{"Nix", "clear"}, "string"=w573:string)  [unwired: 9 in]
            n266 = case shown="\"clear\"" w570 {
              tunnel: w572 -> [w575 w578]
              tunnel: [w575 w577] -> w571
              frame "Nix", Default {
              }
              frame "clear" {
                n267 = Enqueue Element(queue=w578, element="cline") -> (queue out=w577:refnum<queue>)  [unwired: 2 in, 2 out]
              }
            }
            n268 = Enqueue Element(queue=w571, element=w573) -> ()  [unwired: 2 in, 3 out]
          }
        }
        n269 = event-data("Discard?"=w558) -> ()  [unwired: 1 in, 1 out]
      }
    }
  }
  n270 = property on="L" class="WFGraph (strict)"("Active Cursor"=u32 0, "Cursor.Cursor X"=10.0 ("Cursor.Cursor Position:Cursor X"), "Active Cursor"=u32 1, "Cursor.Cursor X"=90.0 ("Cursor.Cursor Position:Cursor X")) -> ()  [unwired: 2 in, 2 out]
  n271 = property on="a" class="WFGraph (strict)"("Active Cursor"=u32 0, "Cursor.Cursor X"=-40.0 ("Cursor.Cursor Position:Cursor X"), "Active Cursor"=u32 1, "Cursor.Cursor X"=40.0 ("Cursor.Cursor Position:Cursor X")) -> ()  [unwired: 2 in, 2 out]
  n272 = property on="b" class="WFGraph (strict)"("Active Cursor"=u32 0, "Cursor.Cursor X"=-40.0 ("Cursor.Cursor Position:Cursor X"), "Active Cursor"=u32 1, "Cursor.Cursor X"=40.0 ("Cursor.Cursor Position:Cursor X")) -> ()  [unwired: 2 in, 2 out]
